vi "泵压力标定.vi"(11 "振动泵信号输入":dbl) -> (3 "振动泵压力输出":dbl)   [LabVIEW 2016]
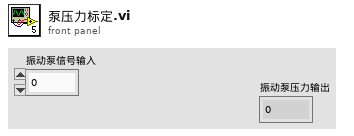
[diagram p1: front panel]
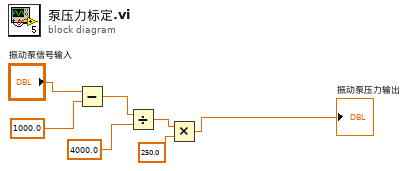
[diagram p0: block diagram]
diagram:
  n1 = Subtract(x="振动泵信号输入", y=1000.0) -> (x-y=w5:dbl)
  n2 = Divide(x=w5, y=4000.0) -> (x/y=w3:dbl)
  n3 = Multiply(x=w3, y=250.0) -> (x*y=→"振动泵压力输出":dbl)
